vi "SSL_Disconnect.vi"(8 "error in (no error)":errorcluster, 11 "SSL_Connection":T1) -> (0 "error out":errorcluster)   [LabVIEW 2018, in "AWS_IoT.lvlib"]
doc: "MIT License\n\nCopyright (c) 2016 Indie-Energy\n\nPermission is hereby granted, free of charge, to any person obtaining a copy\nof this software and associated documentation files (the \"Software\"), to deal\nin the Software without restriction, including without limitation the rights\nto use, copy, modify, merge, publish, distribute, sublicense, and/or sell\ncopies of the Software, and to permit persons to whom the Software is\nfurnished to do so, subject to the following conditions:\n\nThe above copyright notice and this permission notice shall be included in all\ncopies or substantial portions of the Software.\n\nTHE SOFTWARE IS PROVIDED \"AS IS\", WITHOUT WARRANTY OF ANY KIND, EXPRESS OR\nIMPLIED, INCLUDING BUT NOT LIMITED TO THE WARRANTIES OF MERCHANTABILITY,\nFITNESS FOR A PARTICULAR PURPOSE AND NONINFRINGEMENT. IN NO EVENT SHALL THE\nAUTHORS OR COPYRIGHT HOLDERS BE LIABLE FOR ANY CLAIM, DAMAGES OR OTHER\nLIABILITY, WHETHER IN AN ACTION OF CONTRACT, TORT OR OTHERWISE, ARISING FROM,\nOUT OF OR IN CONNECTION WITH THE SOFTWARE OR THE USE OR OTHER DEALINGS IN THE\nSOFTWARE."
uses:
  AWS_IoT.lvlib
  Controls/SSL_Connection.ctl
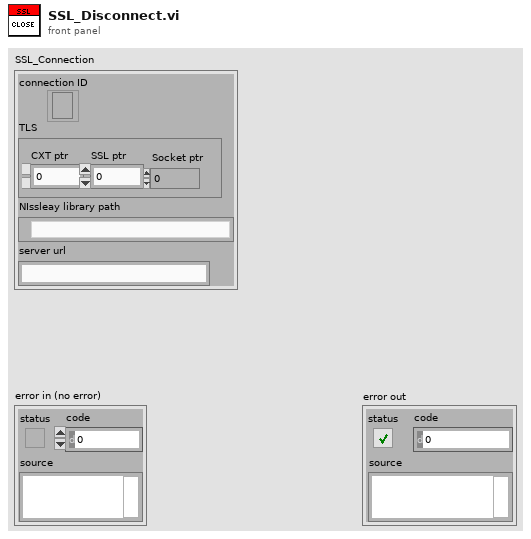
[diagram p1: front panel]
types:
  T1 = typedef "AWS_IoT.lvlib/SSL_Connection.ctl" = cluster{"connection ID":refnum<k5>, "TLS":cluster{"CXT ptr":i32, "SSL ptr":i32, "Socket ptr":i32}, "NIssleay library path":path, "server url":string}
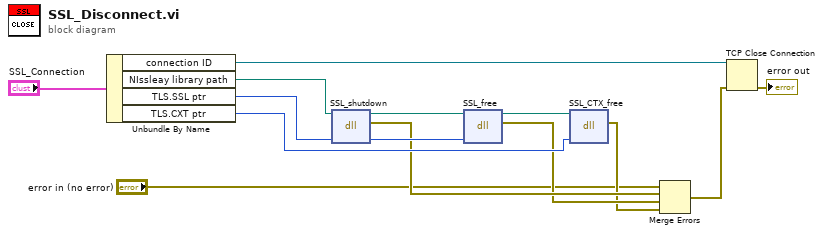
[diagram p0: block diagram]
diagram:
  n1 = Unbundle By Name("SSL_Connection") -> ("connection ID"=w4:refnum<k5>, "NIssleay library path"=w1:path, "TLS.SSL ptr"=w10:i32, "TLS.CXT ptr"=w9:i32)
  n2 = dll-call lib="NIssleay32.*" fn="SSL_shutdown"(path in=w1, "SSL"=w10) -> (path out=w12:path, error out=w8:errorcluster, "SSL"=w11:i32)  [unwired: 3 in]
  n3 = dll-call lib="NIssleay32.*" fn="SSL_free"(path in=w12, "SSL"=w11) -> (path out=w13:path, error out=w7:errorcluster)  [unwired: 4 in]
  n4 = dll-call lib="NIssleay32.*" fn="SSL_CTX_free"(path in=w13, "Context"=w9) -> (error out=w6:errorcluster)  [unwired: 4 in, 1 out]
  n5 = Merge Errors("error in (no error)", w8, w7, w6) -> (w3:errorcluster)
  n6 = TCP Close Connection(connection ID=w4, error in (no error)=w3) -> (error out=→"error out":errorcluster)  [unwired: 1 in, 1 out]
